vi "Read_From_Dashboard.vi"   [LabVIEW 2018]
uses:
  <vilib>/Rock Robotics/Network Tables/NT Read Number.vi
  Global_Variables/Dashboard_Globals.vi
  <vilib>/Rock Robotics/Network Tables/NT Read String.vi
  <vilib>/Rock Robotics/Network Tables/NT Read Boolean.vi
  Global_Variables/Drive_Globals.vi
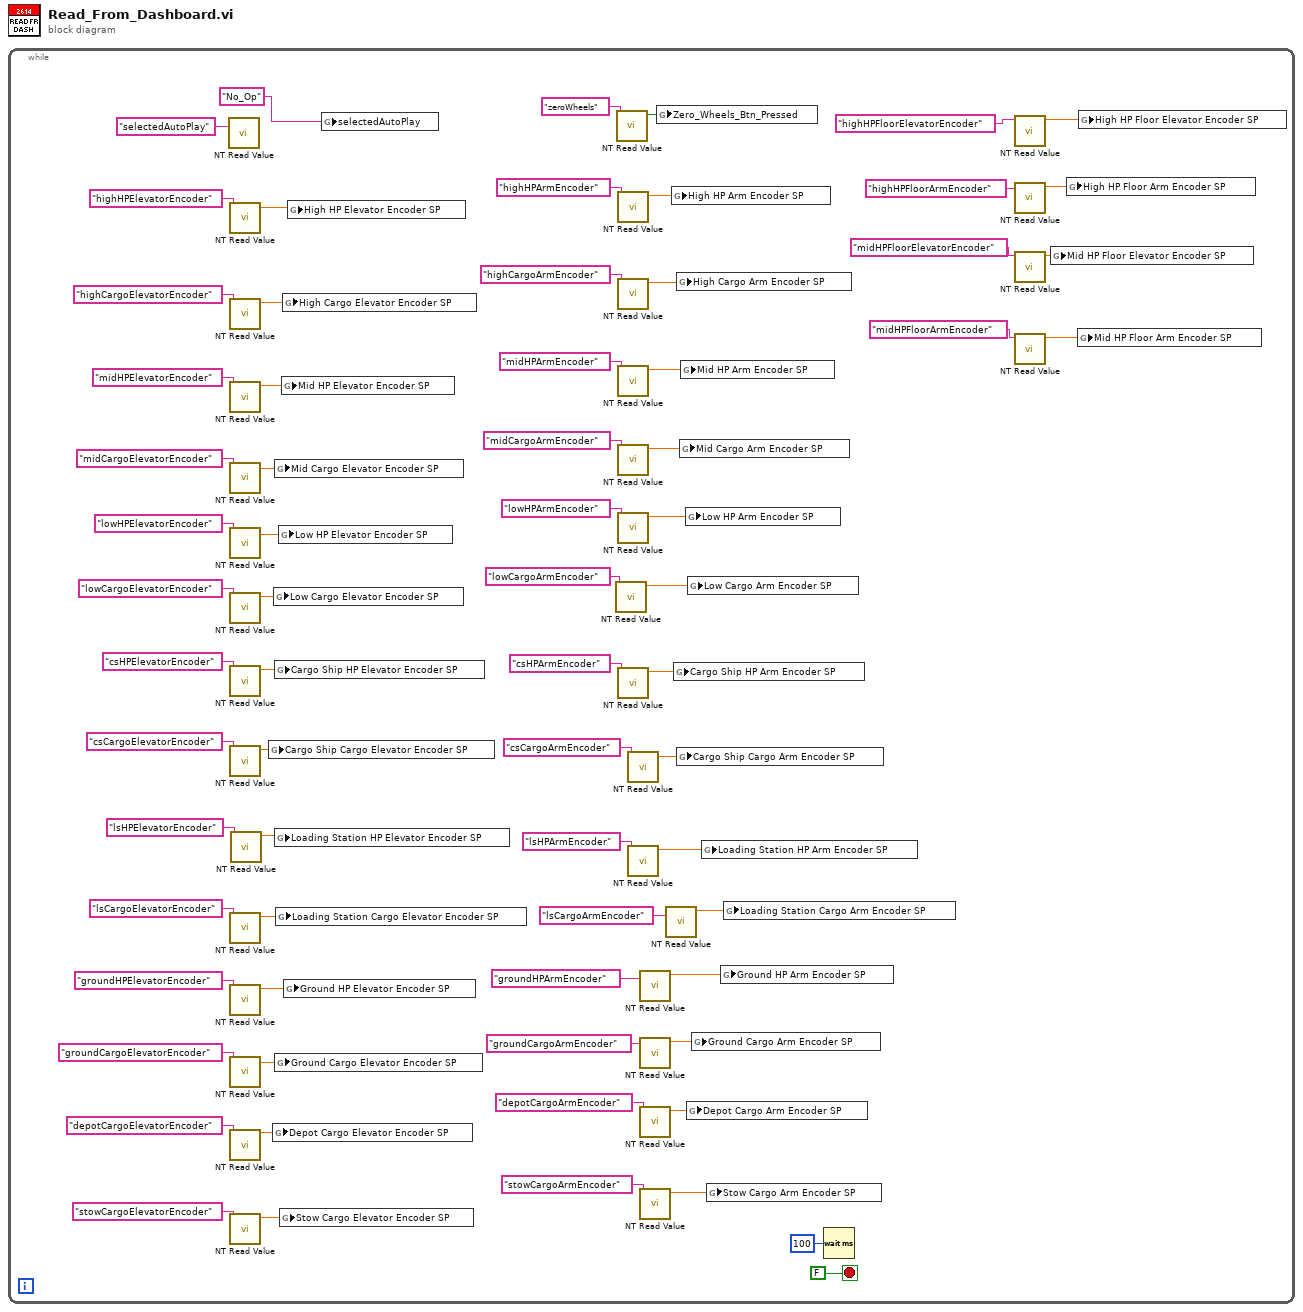
[diagram p0: block diagram]
diagram:
  n1 = while {
    stop <- FALSE stop-if-true
    n2 = call-poly <vilib>:"NT Read Value.vi"("Name"="selectedAutoPlay") -> ()  [unwired: 9 in, 2 out]
    n3 = call-poly <vilib>:"NT Read Value.vi"("Name"="highHPElevatorEncoder") -> ("Numeric"=w39:dbl)  [unwired: 9 in, 1 out]
    n4 = call-poly <vilib>:"NT Read Value.vi"("Name"="highCargoElevatorEncoder") -> ("Numeric"=w38:dbl)  [unwired: 9 in, 1 out]
    n5 = call-poly <vilib>:"NT Read Value.vi"("Name"="midHPElevatorEncoder") -> ("Numeric"=w34:dbl)  [unwired: 9 in, 1 out]
    n6 = call-poly <vilib>:"NT Read Value.vi"("Name"="midCargoElevatorEncoder") -> ("Numeric"=w30:dbl)  [unwired: 9 in, 1 out]
    n7 = call-poly <vilib>:"NT Read Value.vi"("Name"="lowHPElevatorEncoder") -> ("Numeric"=w29:dbl)  [unwired: 9 in, 1 out]
    n8 = call-poly <vilib>:"NT Read Value.vi"("Name"="lowCargoElevatorEncoder") -> ("Numeric"=w28:dbl)  [unwired: 9 in, 1 out]
    n9 = call-poly <vilib>:"NT Read Value.vi"("Name"="csHPElevatorEncoder") -> ("Numeric"=w27:dbl)  [unwired: 9 in, 1 out]
    n10 = call-poly <vilib>:"NT Read Value.vi"("Name"="csCargoElevatorEncoder") -> ("Numeric"=w25:dbl)  [unwired: 9 in, 1 out]
    n11 = call-poly <vilib>:"NT Read Value.vi"("Name"="lsCargoElevatorEncoder") -> ("Numeric"=w20:dbl)  [unwired: 9 in, 1 out]
    n12 = call-poly <vilib>:"NT Read Value.vi"("Name"="groundHPElevatorEncoder") -> ("Numeric"=w19:dbl)  [unwired: 9 in, 1 out]
    n13 = call-poly <vilib>:"NT Read Value.vi"("Name"="groundCargoElevatorEncoder") -> ("Numeric"=w16:dbl)  [unwired: 9 in, 1 out]
    n14 = call-poly <vilib>:"NT Read Value.vi"("Name"="depotCargoElevatorEncoder") -> ("Numeric"=w15:dbl)  [unwired: 9 in, 1 out]
    n15 = call-poly <vilib>:"NT Read Value.vi"("Name"="stowCargoElevatorEncoder") -> ("Numeric"=w13:dbl)  [unwired: 9 in, 1 out]
    n16 = call-poly <vilib>:"NT Read Value.vi"("Name"="lsHPElevatorEncoder") -> ("Numeric"=w23:dbl)  [unwired: 9 in, 1 out]
    n17 = global write "Dashboard_Globals.vi" "Cargo Ship Cargo Elevator Encoder SP"(w25) -> ()
    n18 = global write "Dashboard_Globals.vi" "Depot Cargo Elevator Encoder SP"(w15) -> ()
    n19 = global write "Dashboard_Globals.vi" "Low Cargo Elevator Encoder SP"(w28) -> ()
    n20 = global write "Dashboard_Globals.vi" "Mid Cargo Elevator Encoder SP"(w30) -> ()
    n21 = global write "Dashboard_Globals.vi" "Cargo Ship HP Elevator Encoder SP"(w27) -> ()
    n22 = global write "Dashboard_Globals.vi" "Loading Station HP Elevator Encoder SP"(w23) -> ()
    n23 = global write "Dashboard_Globals.vi" "Ground Cargo Elevator Encoder SP"(w16) -> ()
    n24 = global write "Dashboard_Globals.vi" "Loading Station Cargo Elevator Encoder SP"(w20) -> ()
    n25 = global write "Dashboard_Globals.vi" "Low HP Elevator Encoder SP"(w29) -> ()
    n26 = global write "Dashboard_Globals.vi" "Stow Cargo Elevator Encoder SP"(w13) -> ()
    n27 = global write "Dashboard_Globals.vi" "Mid HP Elevator Encoder SP"(w34) -> ()
    n28 = global write "Dashboard_Globals.vi" "High Cargo Elevator Encoder SP"(w38) -> ()
    n29 = global write "Dashboard_Globals.vi" "Ground HP Elevator Encoder SP"(w19) -> ()
    n30 = global write "Dashboard_Globals.vi" "High HP Elevator Encoder SP"(w39) -> ()
    n31 = global write "Dashboard_Globals.vi" "selectedAutoPlay"("No_Op" ("Name")) -> ()
    n32 = call-poly <vilib>:"NT Read Value.vi"("Name"="lowCargoArmEncoder") -> ("Numeric"=w31:dbl)  [unwired: 9 in, 1 out]
    n33 = call-poly <vilib>:"NT Read Value.vi"("Name"="zeroWheels") -> ("Boolean"=w10:bool)  [unwired: 9 in, 1 out]
    n34 = call-poly <vilib>:"NT Read Value.vi"("Name"="highHPArmEncoder") -> ("Numeric"=w37:dbl)  [unwired: 9 in, 1 out]
    n35 = call-poly <vilib>:"NT Read Value.vi"("Name"="highCargoArmEncoder") -> ("Numeric"=w36:dbl)  [unwired: 9 in, 1 out]
    n36 = call-poly <vilib>:"NT Read Value.vi"("Name"="midHPArmEncoder") -> ("Numeric"=w35:dbl)  [unwired: 9 in, 1 out]
    n37 = call-poly <vilib>:"NT Read Value.vi"("Name"="midCargoArmEncoder") -> ("Numeric"=w33:dbl)  [unwired: 9 in, 1 out]
    n38 = call-poly <vilib>:"NT Read Value.vi"("Name"="lowHPArmEncoder") -> ("Numeric"=w32:dbl)  [unwired: 9 in, 1 out]
    n39 = call-poly <vilib>:"NT Read Value.vi"("Name"="csHPArmEncoder") -> ("Numeric"=w26:dbl)  [unwired: 9 in, 1 out]
    n40 = call-poly <vilib>:"NT Read Value.vi"("Name"="csCargoArmEncoder") -> ("Numeric"=w24:dbl)  [unwired: 9 in, 1 out]
    n41 = call-poly <vilib>:"NT Read Value.vi"("Name"="lsHPArmEncoder") -> ("Numeric"=w22:dbl)  [unwired: 9 in, 1 out]
    n42 = call-poly <vilib>:"NT Read Value.vi"("Name"="groundHPArmEncoder") -> ("Numeric"=w18:dbl)  [unwired: 9 in, 1 out]
    n43 = call-poly <vilib>:"NT Read Value.vi"("Name"="groundCargoArmEncoder") -> ("Numeric"=w17:dbl)  [unwired: 9 in, 1 out]
    n44 = call-poly <vilib>:"NT Read Value.vi"("Name"="depotCargoArmEncoder") -> ("Numeric"=w14:dbl)  [unwired: 9 in, 1 out]
    n45 = call-poly <vilib>:"NT Read Value.vi"("Name"="stowCargoArmEncoder") -> ("Numeric"=w12:dbl)  [unwired: 9 in, 1 out]
    n46 = global write "Drive_Globals.vi" "Zero_Wheels_Btn_Pressed"(w10) -> ()
    n47 = call-poly <vilib>:"NT Read Value.vi"("Name"="lsCargoArmEncoder") -> ("Numeric"=w21:dbl)  [unwired: 9 in, 1 out]
    n48 = global write "Dashboard_Globals.vi" "High HP Arm Encoder SP"(w37) -> ()
    n49 = global write "Dashboard_Globals.vi" "Cargo Ship HP Arm Encoder SP"(w26) -> ()
    n50 = global write "Dashboard_Globals.vi" "High Cargo Arm Encoder SP"(w36) -> ()
    n51 = global write "Dashboard_Globals.vi" "Cargo Ship Cargo Arm Encoder SP"(w24) -> ()
    n52 = global write "Dashboard_Globals.vi" "Mid Cargo Arm Encoder SP"(w33) -> ()
    n53 = global write "Dashboard_Globals.vi" "Mid HP Arm Encoder SP"(w35) -> ()
    n54 = global write "Dashboard_Globals.vi" "Low HP Arm Encoder SP"(w32) -> ()
    n55 = global write "Dashboard_Globals.vi" "Depot Cargo Arm Encoder SP"(w14) -> ()
    n56 = global write "Dashboard_Globals.vi" "Low Cargo Arm Encoder SP"(w31) -> ()
    n57 = global write "Dashboard_Globals.vi" "Ground Cargo Arm Encoder SP"(w17) -> ()
    n58 = global write "Dashboard_Globals.vi" "Loading Station HP Arm Encoder SP"(w22) -> ()
    n59 = global write "Dashboard_Globals.vi" "Stow Cargo Arm Encoder SP"(w12) -> ()
    n60 = global write "Dashboard_Globals.vi" "Ground HP Arm Encoder SP"(w18) -> ()
    n61 = global write "Dashboard_Globals.vi" "Loading Station Cargo Arm Encoder SP"(w21) -> ()
    n62 = Wait (ms)(milliseconds to wait=u32 100) -> ()  [unwired: 1 out]
    n63 = call-poly <vilib>:"NT Read Value.vi"("Name"="highHPFloorElevatorEncoder") -> ("Numeric"=w9:dbl)  [unwired: 9 in, 1 out]
    n64 = call-poly <vilib>:"NT Read Value.vi"("Name"="highHPFloorArmEncoder") -> ("Numeric"=w8:dbl)  [unwired: 9 in, 1 out]
    n65 = call-poly <vilib>:"NT Read Value.vi"("Name"="midHPFloorElevatorEncoder") -> ("Numeric"=w7:dbl)  [unwired: 9 in, 1 out]
    n66 = call-poly <vilib>:"NT Read Value.vi"("Name"="midHPFloorArmEncoder") -> ("Numeric"=w6:dbl)  [unwired: 9 in, 1 out]
    n67 = global write "Dashboard_Globals.vi" "Mid HP Floor Elevator Encoder SP"(w7) -> ()
    n68 = global write "Dashboard_Globals.vi" "High HP Floor Arm Encoder SP"(w8) -> ()
    n69 = global write "Dashboard_Globals.vi" "Mid HP Floor Arm Encoder SP"(w6) -> ()
    n70 = global write "Dashboard_Globals.vi" "High HP Floor Elevator Encoder SP"(w9) -> ()
  }
